vi "3-3.vi"(0 "字符串":string, 1 "C 6":dbl, 2 "C":dbl, 3 "U":dbl, 4 "数值 3":dbl, 5 "A 5":dbl) -> (6 "字符串 2":string, 7 "字符串 3":string, 8 "数值 4":dbl)   [LabVIEW 2017]
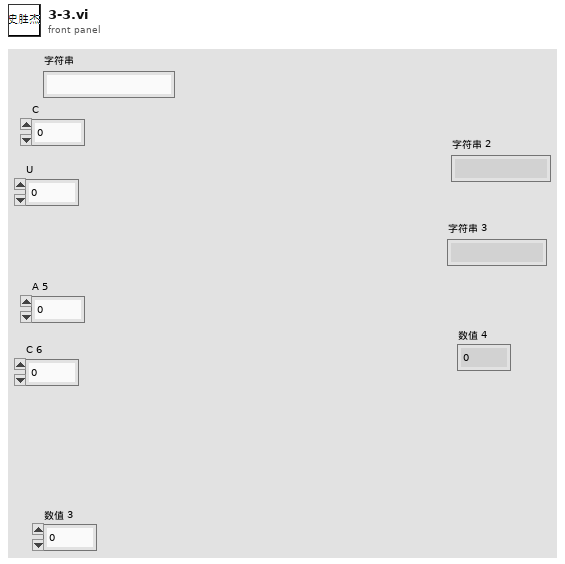
[diagram p1: front panel]
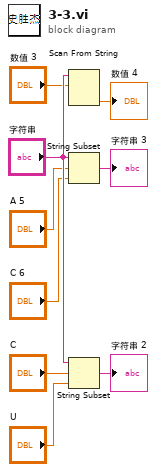
[diagram p0: block diagram]
diagram:
  n1 = Scan From String(input string="字符串", initial scan location="数值 3") -> (output 1=→"数值 4":dbl)  [unwired: 3 in, 3 out]
  n2 = String Subset(string="字符串", offset (0)="A 5", length (rest)="C 6") -> (substring=→"字符串 3":string)
  n3 = String Subset(string="字符串", offset (0)="C", length (rest)="U") -> (substring=→"字符串 2":string)
